vi "CoboltLaser_Example_LaserStatusBasicGet.vi"(0 "ComPort":refnum<visa-resource-name>, 7 "error in (no error)":errorcluster) -> (27 "error out":errorcluster)   [LabVIEW 2012, in "Cobolt.lvclass"]
uses:
  Template/Cobolt.lvclass
panel:
  out "OperatingHours":dbl
  out "Fault":string
  out "Error":bool
  out "LaserLock":bool
  out "LaserOn":bool
  out "PowerOn":bool
  out "SerialNumber":string
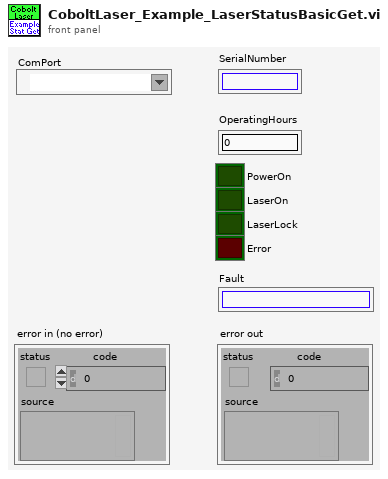
[diagram p1: front panel]
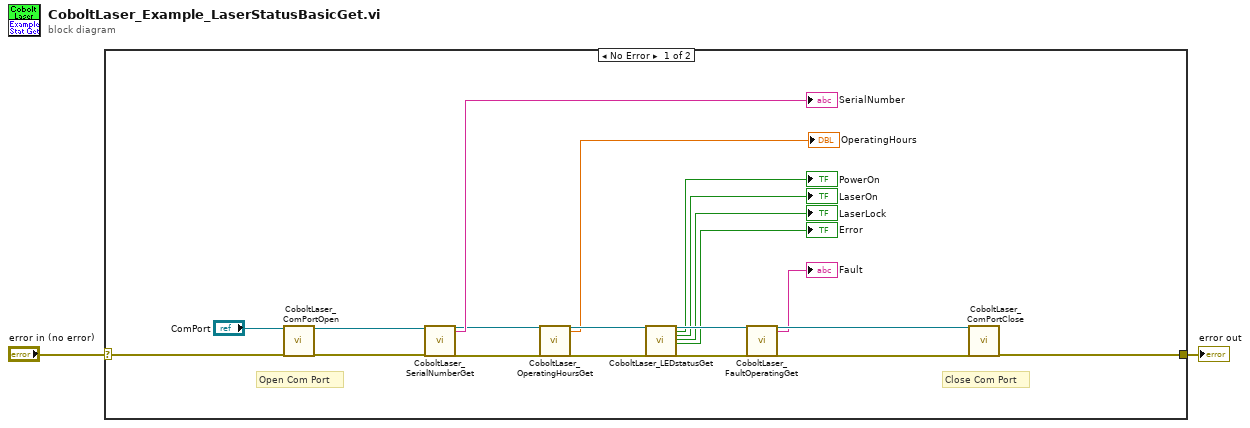
[diagram p0: block diagram]
diagram:
  n1 = case shown="No Error" "error in (no error)" {
    selector: "error in (no error)" -> [w22 w23]
    tunnel: [w18 w23] -> w1
    frame No Error {
      # "Close Com Port"
      # "Open Com Port"
      n2 = call "CoboltLaser_ComPortOpen.vi"("ComPort"="ComPort", "error in (no error)"=w22) -> ("ComPort Out"=w16:refnum<visa-resource-name>, "error out"=w21:errorcluster)  [unwired: 16 in]
      n3 = call "CoboltLaser_SerialNumberGet.vi"("ComPort"=w16, "error in (no error)"=w21) -> ("ComPortOut"=w5:refnum<visa-resource-name>, "SerialNumber"=→"SerialNumber":string, "error out"=w7:errorcluster)  [unwired: 23 in]
      n4 = call "CoboltLaser_OperatingHoursGet.vi"("ComPort"=w5, "error in (no error)"=w7) -> ("ComPortOut"=w4:refnum<visa-resource-name>, "OperatingHours"=→"OperatingHours":dbl, "error out"=w6:errorcluster)  [unwired: 23 in]
      n5 = call "CoboltLaser_LEDstatusGet.vi"("ComPort"=w4, "error in (no error)"=w6) -> ("ComPortOut"=w15:refnum<visa-resource-name>, "PowerOn"=→"PowerOn":bool, "LaserOn"=→"LaserOn":bool, "LaserLock"=→"LaserLock":bool, "Error"=→"Error":bool, "error out"=w20:errorcluster)  [unwired: 20 in]
      n6 = call "CoboltLaser_FaultOperatingGet.vi"("ComPort"=w15, "error in (no error)"=w20) -> ("ComPortOut"=w14:refnum<visa-resource-name>, "Fault"=→"Fault":string, "error out"=w19:errorcluster)  [unwired: 23 in]
      n7 = call "CoboltLaser_ComPortClose.vi"("ComPort"=w14, "error in (no error)"=w19) -> ("error out"=w18:errorcluster)  [unwired: 17 in]
    }
    frame Error {
    }
  }
  "error out" <- w1
